vi "Get All Sequence Names.vi"(8 "error in (no error)":errorcluster, 11 "Session Ref in":T1) -> (0 "error out":errorcluster, 2 "Sequence Names out":string[](array[string]), 3 "Session Ref out":T1)   [LabVIEW 2020, in "NI_VS Sequence Execution Interface.lvlib"]
doc: "Returns a list of sequence names for all the real-time sequences in an NI VeriStand stimulus profile session."
uses:
  <vilib>/NI VeriStand/Execution/SequenceExecutionInterface/NI_VS Sequence Execution Interface.lvlib
  <vilib>/NI VeriStand/Execution/SequenceExecutionInterface/Stimulus Profile Session Ref.ctl
  NationalInstruments.VeriStand.ClientAPI
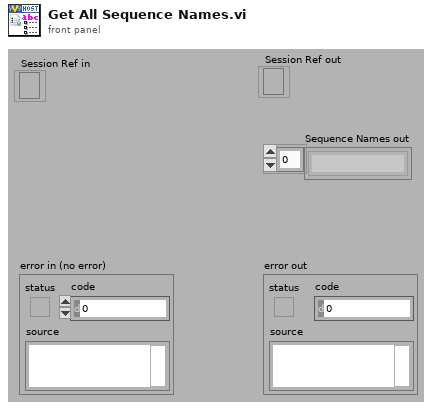
[diagram p1: front panel]
types:
  T1 = typedef "NI_VS Sequence Execution Interface.lvlib/Stimulus Profile Session Ref.ctl" = refnum<k24>
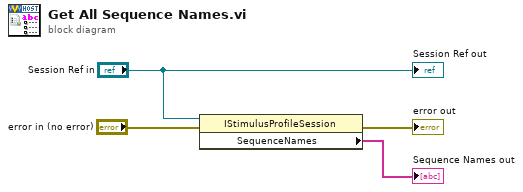
[diagram p0: block diagram]
diagram:
  n1 = property class="IStimulusProfileSession"(reference="Session Ref in", error in="error in (no error)") -> (error out=→"error out":errorcluster, "SequenceNames"=→"Sequence Names out":string[])  [unwired: 1 out]
  "Session Ref out" <- "Session Ref in"
